vi "dfd_Get SOS TFs.vi"(8 "error in (no error)":errorcluster, 11 "filter coef":T1) -> (0 "error out":errorcluster, 2 "dens":dbl[][](array[numeric]), 3 "nums":dbl[][](array[numeric]), 5 "gain":dbl)   [LabVIEW 2017, in "NI_DigFilterLicensed.lvlib"]
uses:
  <vilib>/addons/Digital Filter Design/NI_DigFilterLicensed.lvlib
  <vilib>/addons/Digital Filter Design/_Objects.llb/DFD Filter Coef.ctl
  <vilib>/addons/Digital Filter Design/_Objects.llb/DFD Filter Structure Type Selector.ctl
panel:
  out "#sec":i32
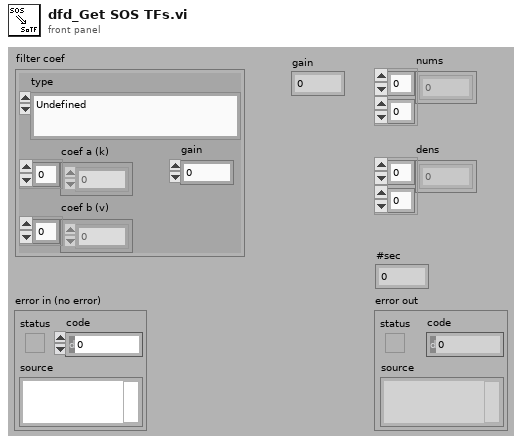
[diagram p1: front panel]
types:
  T1 = typedef "NI_DigFilterLicensed.lvlib/DFD Filter Coef.ctl" = cluster{"type":T2, "gain":dbl, "coef a (k)":dbl[], "coef b (v)":dbl[]}
  T2 = typedef "NI_DigFilterLicensed.lvlib/DFD Filter Structure Type Selector.ctl" = enum16{"Undefined", "FIR Direct Form", "FIR Direct Form Transposed", "FIR Symmetric", "FIR Antisymmetric", "IIR Direct Form I", "IIR Direct Form I Transposed", "IIR Direct Form II", "IIR Direct Form II Transposed", "IIR Cascaded Second Order Sections Form I", "IIR Cascaded Second Order Sections Form I Transposed", "IIR Cascaded Second Order Sections Form II", "IIR Cascaded Second Order Sections Form II Transposed", "Lattice Allpass (basic sections)", "Lattice Allpass (one multiplier sections)", "Lattice Allpass (normalized sections)", "Lattice AR (basic sections)", "Lattice AR (one multiplier sections)", "Lattice AR (normalized sections)", "Lattice MA (minimum phase)", "Lattice MA (maximum phase)", "Lattice ARMA (basic sections)", "Lattice ARMA (one multiplier sections)", "Lattice ARMA (normalized sections)"}
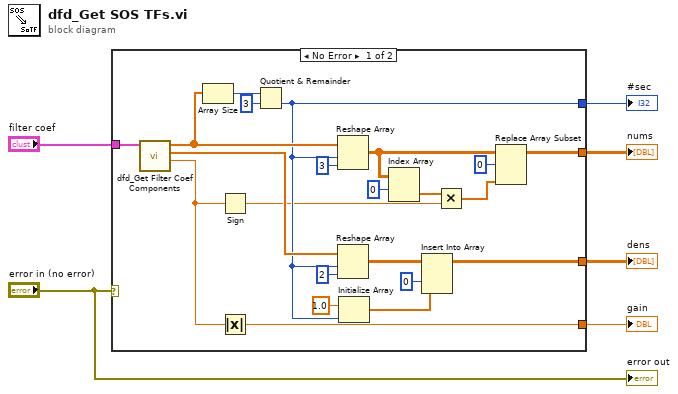
[diagram p0: block diagram]
diagram:
  n1 = case shown="No Error" "error in (no error)" {
    tunnel: "filter coef" -> [w28 _]
    tunnel: [w14 _] -> w5
    tunnel: [w9 _] -> w4
    tunnel: [w21 _] -> w3
    tunnel: [w16 _] -> w2
    frame No Error {
      n2 = call <vilib>:"dfd_Get Filter Coef Components.vi"("filter coef"=w28) -> ("gain"=w8:dbl, "coef a (k)"=w24:dbl[], "coef b (v)"=w25:dbl[])  [unwired: 1 in, 7 out]
      n3 = Array Size(array=w25) -> (size(s)=w27:i32)
      n4 = Sign(1:w8) -> (0:w7:dbl)
      n5 = Absolute Value(x=w8) -> (abs(x)=w14:dbl)
      n6 = Quotient & Remainder(x=w27, y=3) -> (floor(x/y)=w21:i32)  [unwired: 1 out]
      n7 = Reshape Array(w25, w21, 3 ("dimension size")) -> (w12:dbl[][])
      n8 = Reshape Array(w24, w21, 2 ("dimension size")) -> (w19:dbl[][])
      n9 = Initialize Array(1.0 ("element"), w21) -> (w17:dbl[])
      n10 = Index Array(array=w12, index (row)=0) -> (element=w13:dbl[])  [unwired: 1 in]
      n11 = Insert Into Array(array=w19, index (col)=0 ("disabled index (col)"), new element=w17) -> (w16:dbl[][])  [unwired: 1 in]
      n12 = Multiply(x=w13, y=w7) -> (x*y=w10:dbl[])
      n13 = Replace Array Subset(array=w12, new element=w10, index (row)=0) -> (w9:dbl[][])  [unwired: 1 in]
    }
    frame Error {
    }
  }
  "nums" <- w4
  "dens" <- w2
  "gain" <- w5
  "#sec" <- w3
  "error out" <- "error in (no error)"
